vi "TestImageGenerator.vi"() -> ()   [LabVIEW 2011]
panel:
  out "Center of mass":cluster{"comX":sgl, "comY":sgl}
  out "img display":T1(plugin-control)
  in  "y center":dbl=200.0
  in  "x center":dbl=200.0
  in  "spot size":sgl=20.0
  in  "Stop Button":bool
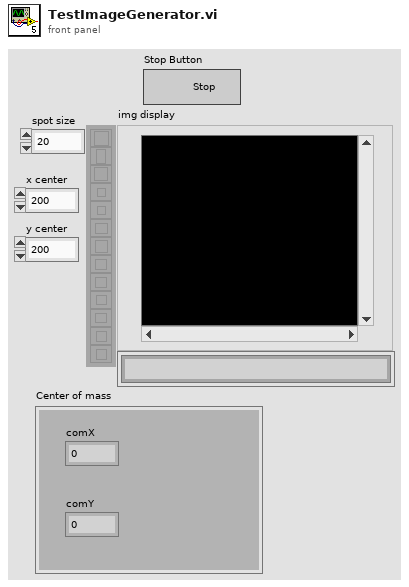
[diagram p1: front panel]
types:
  T1 = typedef "IMAQ Image.ctl" = refnum<image>
  T2 = typedef "Image Type" = u32
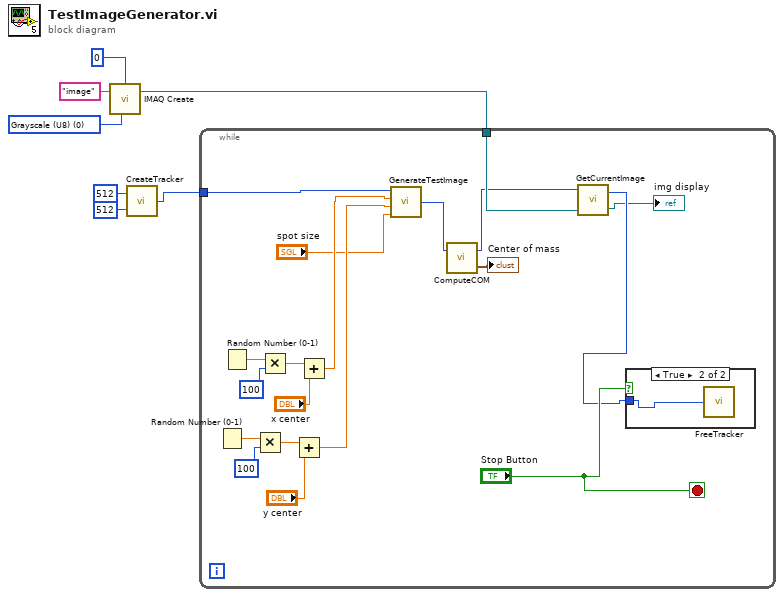
[diagram p0: block diagram]
diagram:
  w3 = T2 0 items=["Grayscale (U8)", "Grayscale (I16)", "Grayscale (SGL)", "Complex (CSG)", "RGB (U32)", "HSL (U32)", "RGB (U64)", "Grayscale (U16)"] ("Image Type")
  n1 = call "IMAQ Create"("Border Size"=0, "Image Name"="image", "Image Type"=w3) -> ("New Image"=w1:T1)  [unwired: 2 in, 1 out]
  n2 = call "CreateTracker.vi"("height"=u32 512, "width"=u32 512) -> ("return type"=w5:u64)
  n3 = while {
    tunnel: w5 -> [w26]
    tunnel: w1 -> [w13]
    stop <- "Stop Button" stop-if-true
    n4 = Random Number (0-1)() -> (number: 0 to 1=w22:dbl)
    n5 = Random Number (0-1)() -> (number: 0 to 1=w25:dbl)
    n6 = Multiply(x=w22, y=100) -> (x*y=w20:dbl)
    n7 = Multiply(x=w25, y=100) -> (x*y=w23:dbl)
    n8 = Add(x=w20, y="y center") -> (x+y=w18:dbl)
    n9 = Add(x=w23, y="x center") -> (x+y=w19:dbl)
    n10 = call "GenerateTestImage.vi"("size"="spot size", "ypos"=w18, "xpos"=w19, "tracker"=w26) -> ("tracker"=w10:u64)
    n11 = call "ComputeCOM.vi"("tracker"=w10) -> ("Center of mass"=→"Center of mass":cluster{"comX":sgl, "comY":sgl}, "tracker"=w8:u64)  [unwired: 1 in]
    n12 = call "GetCurrentImage.vi"("empty image"=w13, "tracker"=w8) -> ("copy of current CUDA image"=→"img display":T1, "tracker"=w12:u64)  [unwired: 1 in]
    n13 = case shown="True" "Stop Button" {
      tunnel: w12 -> [_ w27]
      frame False {
      }
      frame True {
        n14 = call "FreeTracker.vi"("trackerInstance"=w27) -> ()
      }
    }
  }
